vi "Init.vi"(4 "Default Check Value (F)":bool, 6 "Check Value (F)":bool, 7 "Symbols (System Checks)":T1={"Symbol (T - Hover)"=40, "Symbol (F - Hover)"=39, "Symbol (T)"=38, "Symbol (F)"=37}, 8 "error in (no error)":errorcluster, 9 "Enable Cell Editing (F)":bool, 10 "Check All":refnum<vi>, 11 "Multicolumn Listbox":refnum<vi>) -> (0 "error out":errorcluster, 3 "MCListbox with Checkboxes.lvclass":refnum<class "MCListbox with Checkboxes.lvclass">)   [LabVIEW 2016, in "MCListbox with Checkboxes.lvclass"]
uses:
  MCListbox with Checkboxes.lvclass
  MCListbox with Checkboxes.lvclass/MCListbox with Checkboxes.ctl
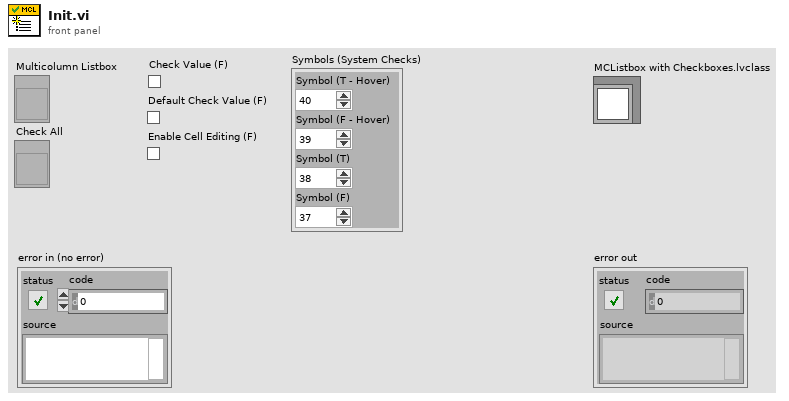
[diagram p1: front panel]
types:
  T1 = cluster{"Symbol (T - Hover)":i32, "Symbol (F - Hover)":i32, "Symbol (T)":i32, "Symbol (F)":i32}
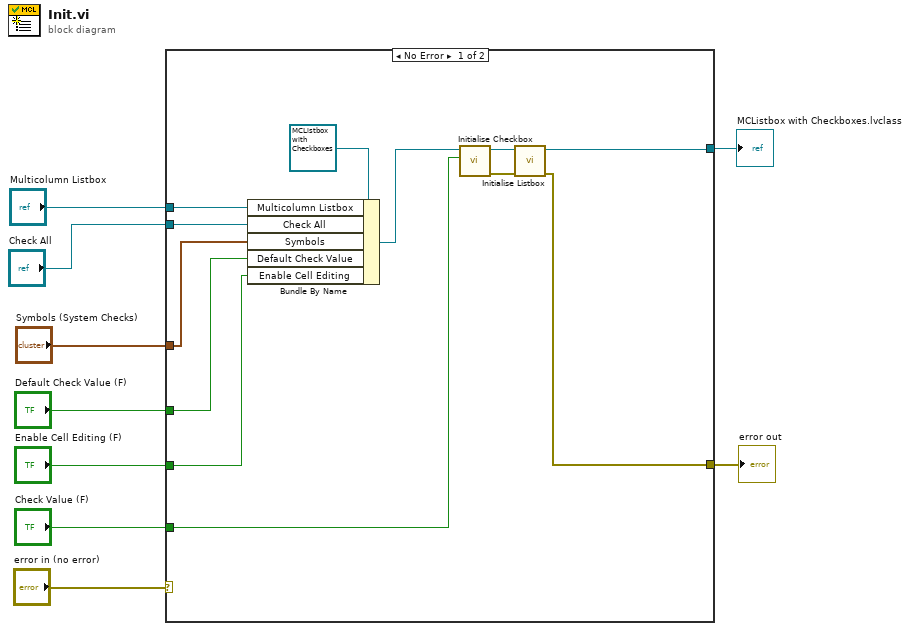
[diagram p0: block diagram]
diagram:
  n1 = case shown="No Error" "error in (no error)" {
    selector: "error in (no error)" -> [_ w22]
    tunnel: [w15 w22] -> w8
    tunnel: [w16 _] -> w7
    tunnel: "Multicolumn Listbox" -> [w20 _]
    tunnel: "Check All" -> [w19 _]
    tunnel: "Check Value (F)" -> [w13 _]
    tunnel: "Symbols (System Checks)" -> [w12 _]
    tunnel: "Default Check Value (F)" -> [w11 _]
    tunnel: "Enable Cell Editing (F)" -> [w10 _]
    frame No Error {
      n2 = Bundle By Name(cluster=refnum<class "MCListbox with Checkboxes.lvclass"> refnum ("MCListbox with Checkboxes.lvclass"), "Multicolumn Listbox"=w20, "Check All"=w19, "Symbols"=w12, "Default Check Value"=w11, "Enable Cell Editing"=w10) -> (w18:refnum<class "MCListbox with Checkboxes.lvclass">)
      n3 = call "Initialise Checkbox.vi"("Check Value (F)"=w13, "MCListbox with Checkboxes in"=w18) -> ("error out"=w14:errorcluster, "MCListbox with Checkboxes out"=w17:refnum<class "MCListbox with Checkboxes.lvclass">)  [unwired: 8 in]
      n4 = call "Initialise Listbox.vi"("error in (no error)"=w14, "MCListbox with Checkboxes in"=w17) -> ("error out"=w15:errorcluster, "MCListbox with Checkboxes out"=w16:refnum<class "MCListbox with Checkboxes.lvclass">)  [unwired: 8 in]
    }
    frame Error {
    }
  }
  "MCListbox with Checkboxes.lvclass" <- w7
  "error out" <- w8
